vi "Add zero.vi"(1 "in":string) -> (0 "out":string)   [LabVIEW 2018]
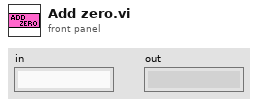
[diagram p1: front panel]
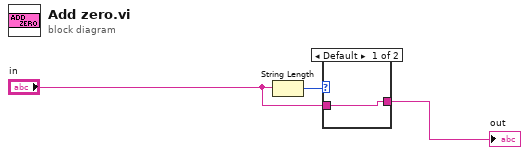
[diagram p0: block diagram]
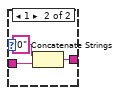
[diagram p2: hidden frame]
diagram:
  n1 = String Length(string="in") -> (length=w1:i32)
  n2 = case shown="Default" w1 {
    tunnel: "in" -> [w4 w6]
    tunnel: [w4 w5] -> w3
    frame Default {
    }
    frame 1 {
      n3 = Concatenate Strings("0" ("string"), w6) -> (w5:string)
    }
  }
  "out" <- w3
